vi "prepDOLT_img.vi"() -> ()   [LabVIEW 2013]
uses:
  <vilib>/DAQmx/write.llb/DAQmx Write (Digital Wfm 1Chan NSamp).vi
  <vilib>/DAQmx/create/channels.llb/DAQmx Create Channel (DO-Digital Output).vi
  <vilib>/DAQmx/configure/timing.llb/DAQmx Timing (Sample Clock).vi
  <vilib>/Waveform/DTblOps.llb/DTbl Boolean Array to Digital.vi
  <vilib>/Waveform/DWDTOps.llb/DWDT Uncompress Digital.vi
  <vilib>/DAQmx/miscellaneous.llb/DAQmx Fill In Error Info.vi
panel:
  in  "number":i32=5
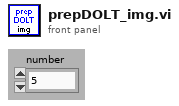
[diagram p1: front panel]
types:
  T1 = cluster{"CH1 AI":tag, "CH1 CI":tag, "CH2 AI":tag, "CH2 CI":tag, "AI X":tag, "AI Y":tag, "AO X-Y":tag, "CH1ST":bool, "CH2ST":bool, "Sigcase":i16, "StageS":i32, "StageL":i32, "data dir":path, "Vp":tag, "Ip":tag, "AO CWlaser":tag, "AO VtoP":tag, "shutter":tag, "LT marker":tag, "488":tag, "532":tag, "640":tag}
  T2 = cluster{"Xpixels":i32, "Vx-min ref":dbl, "Vx-max ref":dbl, "P":dbl, "Ypixels":i32, "Vy-min ref":dbl, "Vy-max ref":dbl, "srate":dbl, "sAOxy":i32, "timeout":dbl, "type":string, "date":string, "time":string, "Colormap":u16, "Drawing Mode":u16, "Scanning Mode":u16, "square pixels":bool, "square matrix":bool, "Xpixels Img":i32, "Vx-min Img":dbl, "VX-max Img":dbl, "Ypixels Img":i32, "Vy-min Img":dbl, "Vy-max Img ":dbl, "Angle Img":dbl, "autoshutter":bool, "finite":bool, "cont":bool, "wavdet":bool, "measpoints":i32, "avpp":i32, "bufferAO":i32, "bufferAI":i32, "CH1":bool, "CH2":bool, "X":bool, "Y":bool, "Ip":bool, "Vp":bool, "starttick":u32, "waveform":path, "Vx-ref":dbl, "Vy-ref":dbl, "refreshrate":dbl, "refreshbuffer":i32, "tt_cycles":i32, "motorref":refnum<k7>, "mirrorswitch":refnum<k7>, "sample mode":i32, "maxbufferAI":i32, "sampletreshold":dbl}
  T3 = cluster{"DOLT":refnum<k21>, "E_DOLT":errorcluster}
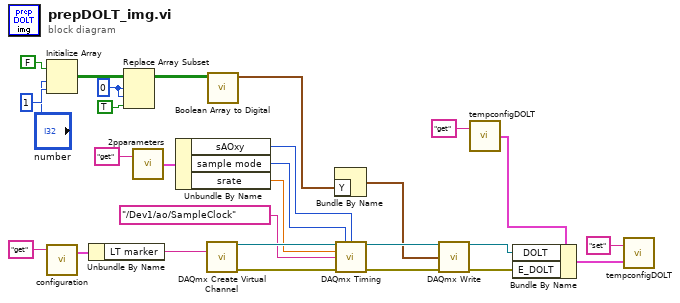
[diagram p0: block diagram]
diagram:
  w6 = 0 ("index")
  n1 = Initialize Array(FALSE, "number", 1 ("dimension size")) -> (w10:bool[][])
  n2 = call "configuration.vi"("command"="get") -> ("config out"=w23:T1)  [unwired: 2 in, 1 out]
  n3 = Unbundle By Name(w23) -> ("LT marker"=w25:tag)
  n4 = Replace Array Subset(array=w10, new element=TRUE, index (row)=w6, index (col)=w6) -> (w5:bool[][])
  n5 = call "2pparameters.vi"("command"="get") -> ("Params out"=w27:T2)  [unwired: 1 in]
  n6 = Unbundle By Name(w27) -> ("sAOxy"=w28:i32, "sample mode"=w13:i32, "srate"=w12:dbl)
  n7 = call-poly <vilib>:"DAQmx Create Virtual Channel.vi"("lines"=w25) -> ("task out"=w16:refnum<k21>, "error out"=w15:errorcluster)  [unwired: 13 in]
  n8 = call-poly <vilib>:"Boolean Array to Digital.vi"("boolean array"=w5) -> ("digital data"=w4:digitaldata)  [unwired: 9 in, 1 out]
  n9 = Bundle By Name("Y"=w4) -> (w11:digitalwaveform)  [unwired: 1 in]
  n10 = call-poly <vilib>:"DAQmx Timing.vi"("task/channels in"=w16, "sample mode"=w13, "samples per channel"=w28, "rate"=w12, "source"=tag "/Dev1/ao/SampleClock", "error in"=w15) -> ("task out"=w22:refnum<k21>, "error out"=w2:errorcluster)  [unwired: 8 in]
  n11 = call-poly <vilib>:"DAQmx Write.vi"("task/channels in"=w22, "data"=w11, "error in"=w2) -> ("task out"=w17:refnum<k21>, "error out"=w1:errorcluster)  [unwired: 10 in, 1 out]
  n12 = call "tempconfigDOLT.vi"("command"="get") -> ("Temp Config out"=w20:T3)  [unwired: 1 in]
  n13 = Bundle By Name(cluster=w20, "DOLT"=w17, "E_DOLT"=w1) -> (w21:T3)
  n14 = call "tempconfigDOLT.vi"("Temp Config in"=w21, "command"="set") -> ()  [unwired: 1 out]
